vi "clock delay.vi"(7 "Delay Time (s)":dbl=1.0 format="%#_13g", 8 "error in (no error)":errorcluster) -> (0 "error out":errorcluster)   [LabVIEW 2019]
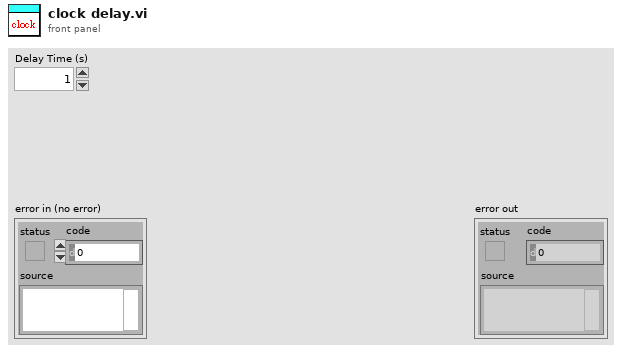
[diagram p1: front panel]
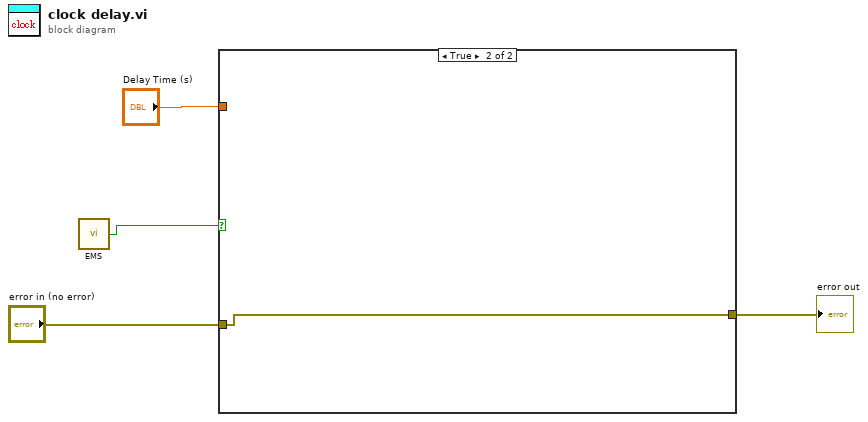
[diagram p0: block diagram]
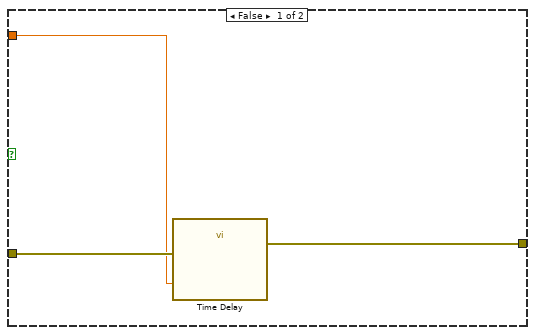
[diagram p2: hidden frame]
diagram:
  n1 = call "EMS.vi"() -> ("A/DIO4 (Pin 19)"=w4:bool)
  n2 = case shown="True" w4 {
    tunnel: "error in (no error)" -> [w7 w8]
    tunnel: [w6 w8] -> w2
    tunnel: "Delay Time (s)" -> [w5 _]
    frame False {
      n3 = call "Time Delay"("error in (no error)"=w7, "Delay Time (s)"=w5) -> ("error out"=w6:errorcluster)  [unwired: 9 in]
    }
    frame True {
    }
  }
  "error out" <- w2
